vi "get_component_type_name.vi"(8 "error in (no error)":errorcluster, 11 "GenericStage in":refnum<class "GenericStage.lvclass">) -> (0 "error out":errorcluster, 2 "component type":string, 3 "GenericStage out":refnum<class "GenericStage.lvclass">)   [LabVIEW 2010, in "GenericStage.lvclass"]
uses:
  GenericStage.lvclass
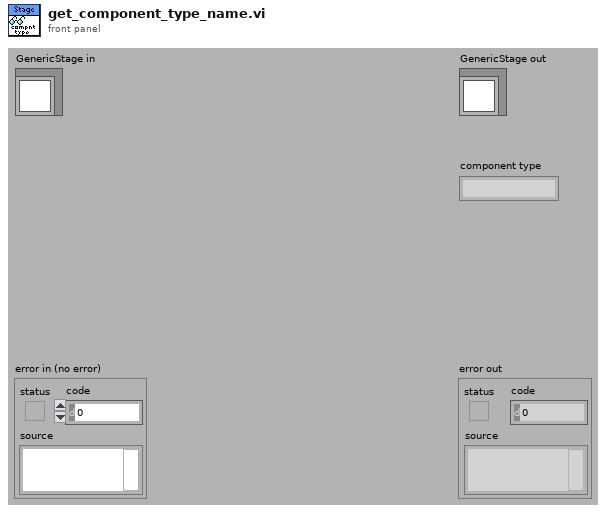
[diagram p1: front panel]
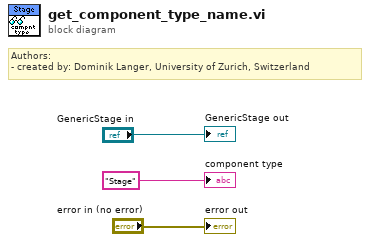
[diagram p0: block diagram]
diagram:
  # "Authors: \n- created by: Dominik Langer, University of Zurich, Switzerland"
  "error out" <- "error in (no error)"
  "GenericStage out" <- "GenericStage in"
  "component type" <- "Stage" ("component type")
